vi "patternDetect.vi"() -> ()   [LabVIEW 2017]
panel:
  out "error out":errorcluster
  in  "error in":errorcluster
  out "Image Out":T1(plugin-control)
  in  "Stop (F)":bool caption="StopCam (F)"
  out "Pattern Class (Particle Classification 1)":string
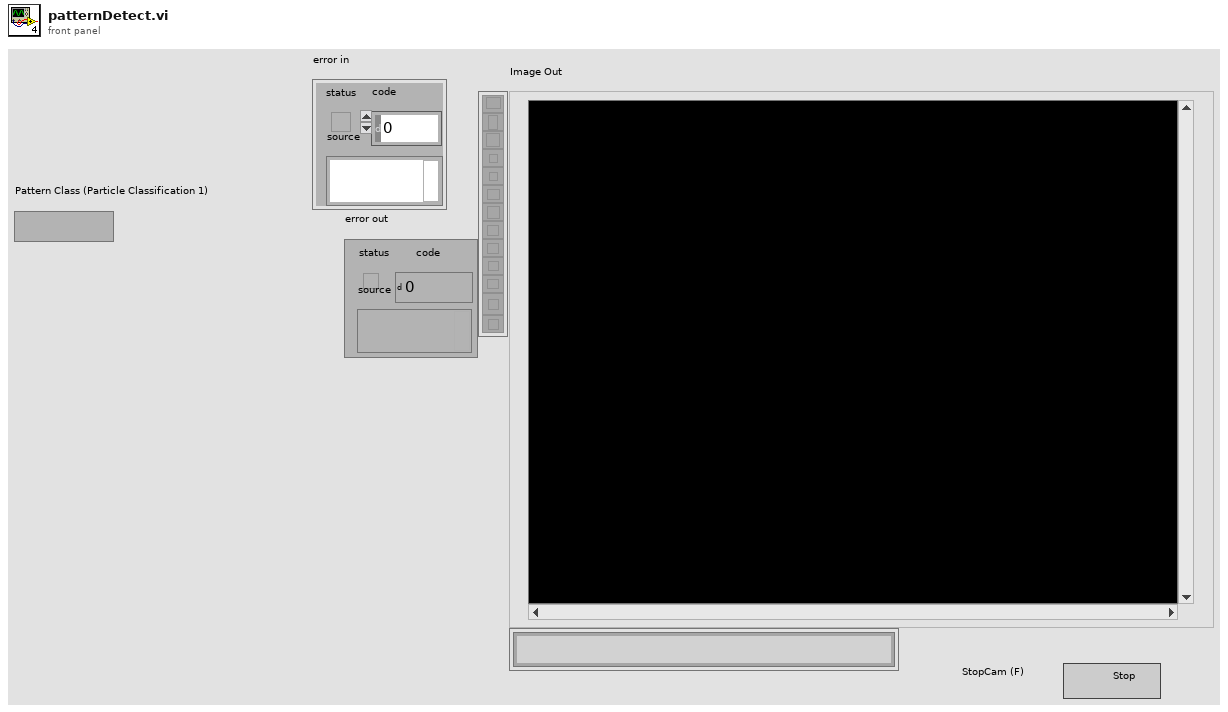
[diagram p1: front panel]
types:
  T1 = typedef "IMAQ Image.ctl" = refnum<image>
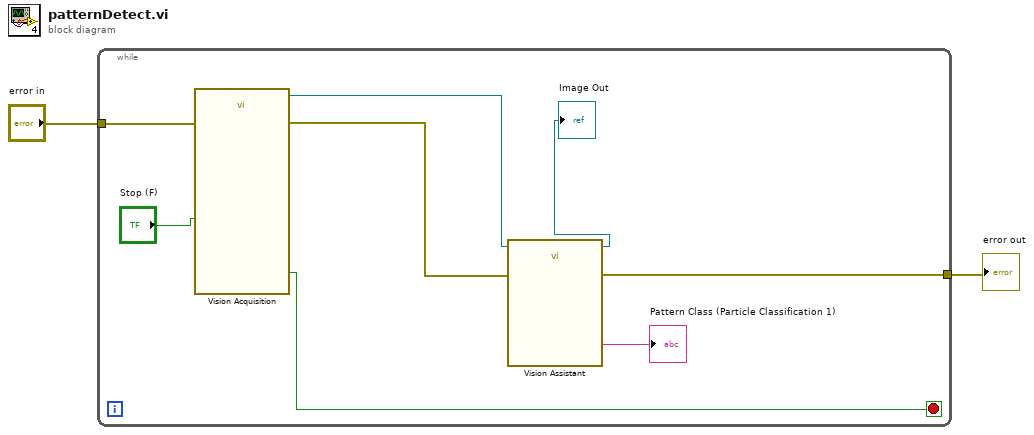
[diagram p0: block diagram]
diagram:
  n1 = while {
    tunnel: "error in" -> [w4]
    tunnel: [w3] -> w1
    stop <- w5 stop-if-true
    n2 = call "Vision Acquisition"("Stop (F)"="Stop (F)", "error in"=w4) -> ("Image Out"=w8:T1, "Stopped"=w5:bool, "error out"=w7:errorcluster)  [unwired: 22 in, 1 out]
    n3 = call "Vision Assistant"("Image In"=w8, "error in"=w7) -> ("Image Out"=→"Image Out":T1, "Class (Particle Classification 1)"=→"Pattern Class (Particle Classification 1)":string, "error out"=w3:errorcluster)  [unwired: 23 in]
  }
  "error out" <- w1
